vi "Write 1Ch 1Samp (I16).vi"(4 "timestamp":timestamp, 6 "index_channel":u32, 8 "error in":errorcluster, 9 "data":i16, 10 "channel":u32, 11 "Writer":refnum<class "Synnax Writer.lvclass">) -> (0 "error out":errorcluster, 3 "Writer Out":refnum<class "Synnax Writer.lvclass">)   [LabVIEW 2026, in "synnax_lib.lvlib" / "Synnax Writer.lvclass"]
uses:
  Synnax Writer.lvclass
  Synnax Writer.lvclass/Synnax Writer.ctl
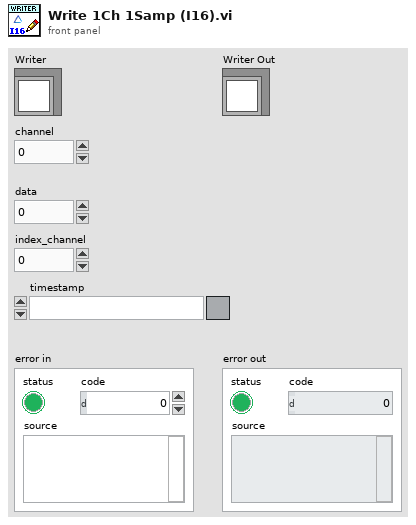
[diagram p1: front panel]
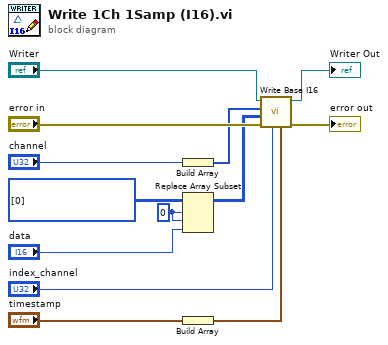
[diagram p0: block diagram]
diagram:
  w7 = 0
  n1 = Build Array("channel") -> (w10:u32[])
  n2 = Replace Array Subset(array=i16[][] [0], new element="data", index (row)=w7, index (col)=w7) -> (w5:i16[][])
  n3 = Build Array("timestamp") -> (w1:timestamp[])
  n4 = call "Write Base I16.vi"("timestamps"=w1, "index_channel"="index_channel", "error in"="error in", "data"=w5, "channels"=w10, "Writer"="Writer") -> ("error out"=→"error out":errorcluster, "Writer Out"=→"Writer Out":refnum<class "Synnax Writer.lvclass">)  [unwired: 4 in]
